vi "Convert C to F.vi"(0 "Display State In":T1, 7 "Degrees Celsius":dbl, 9 "Container State":T2, 11 "error in (no error)":errorcluster) -> (4 "Display State Out":T1, 8 "Degrees Fahrenheit":dbl, 15 "error out":errorcluster)   [LabVIEW 2020, in "Simple Dual Mode Thermometer XControl.xctl"]
doc: "This VI handles the Convert C to F method as part of the Simple Dual Mode Thermometer XControl."
uses:
  Simple Dual Mode Thermometer XControl.xctl
  <vilib>/_xctls/Container State.ctl
  Simple Dual Mode Thermometer State.ctl
  <vilib>/_xctls/XControlSupport.lvlib
panel:
  # "Add Controls & Indicators that form the parameters of the method here. Hook them to the connector pane. Do not delete the controls & indicators that are already hooked to the connector pane.\n\nTo setup the parameters  for this method, right click on this item in the Project Tree & select \"Configure Method...\"."
  # "This simple method converts degrees Celsius to degrees Fahrenheit."
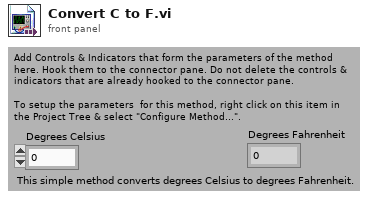
[diagram p1: front panel]
types:
  T1 = typedef "Simple Dual Mode Thermometer XControl.xctl/Simple Dual Mode Thermometer State.ctl" = cluster{"Fahrenheit":bool}
  T2 = typedef "XControlSupport.lvlib/Container State.ctl" = cluster{"Indicator?":bool, "Run Mode?":bool, " Refnum":refnum<vi>}
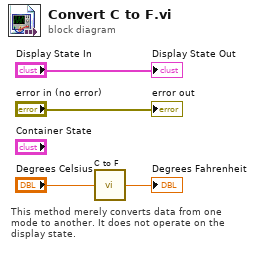
[diagram p0: block diagram]
diagram:
  # "This method merely converts data from one mode to another. It does not operate on the display state."
  n1 = call "C to F.vi"("Celsius"="Degrees Celsius") -> ("Fahrenheit"=→"Degrees Fahrenheit":dbl)
  "Display State Out" <- "Display State In"
  "error out" <- "error in (no error)"
